vi "CRC.vi"(0 "要校验的数组":u8[](array[numeric])) -> (1 "CRC":u16, 2 "CRCHi":u8, 3 "CRCLo":u8)   [LabVIEW 2011]
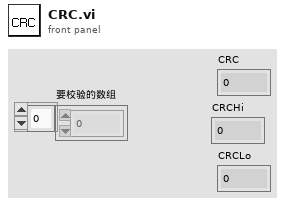
[diagram p1: front panel]
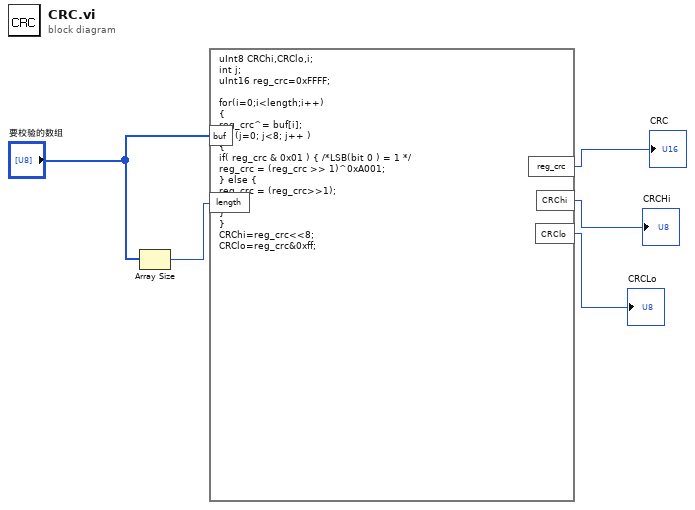
[diagram p0: block diagram]
diagram:
  n1 = Array Size(array="要校验的数组") -> (size(s)=w5:i32)
  n2 = formula code="uInt8 CRChi,CRClo,i;\nint j; \nuInt16 reg_crc=0xFFFF; \n \nfor(i=0;i<length;i++) \n{ \nreg_crc^= buf[i]; \nfor (j=0; j<8; j++ ) \n{ \nif( reg_crc & 0x01 ) { /*LSB(bit 0 ) = 1 */ \nreg_crc = (reg_crc >> 1)^0xA001; \n} else { \nreg_crc = (reg_crc>>1); \n} \n} \n} \nCRChi=reg_crc<<8;\nCRClo=reg_crc&0xff;"("buf"="要校验的数组", "length"=w5) -> ("reg_crc"=→"CRC":u16, "CRChi"=→"CRCHi":u8, "CRClo"=→"CRCLo":u8)
